vi "Init.vi"(8 "error in (no error)":errorcluster, 10 "Init Data":variant, 11 "Cryo Cooler in":refnum<class "Cryo Cooler.lvclass">) -> (0 "error out":errorcluster, 2 "Channel List":refnum<class "HK Item.lvclass">[](array[class]), 3 "Cryo Cooler out":refnum<class "Cryo Cooler.lvclass">)   [LabVIEW 2021, in "Cryo Cooler.lvclass"]
uses:
  Cryo Cooler.lvclass
  hk-channel-class/HK Item/HK Item.lvclass
  Cryo Cooler.lvclass/Cryo Cooler.ctl
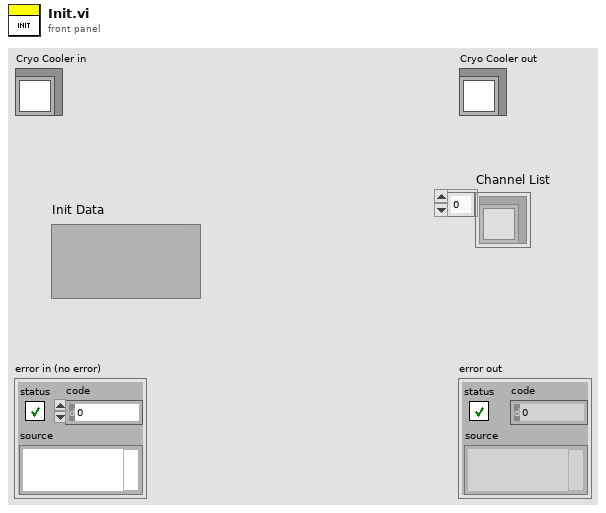
[diagram p1: front panel]
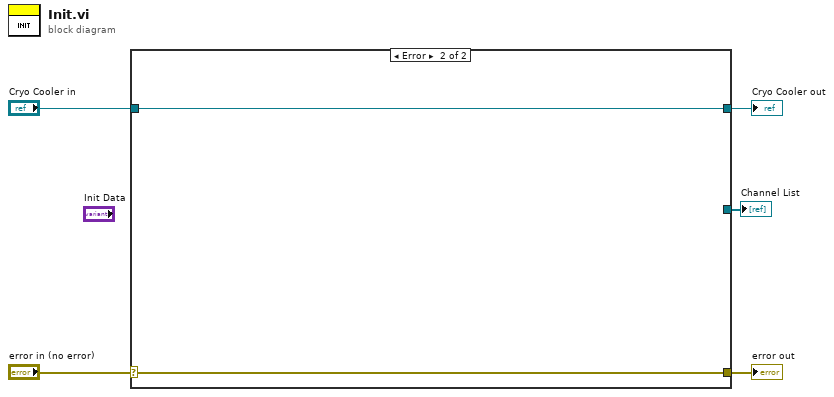
[diagram p0: block diagram]
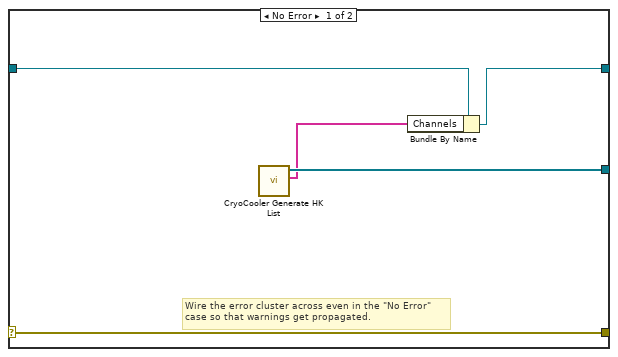
[diagram p2: hidden frame]
diagram:
  n1 = case shown="Error" "error in (no error)" {
    selector: "error in (no error)" -> [w10 w12]
    tunnel: [w10 w12] -> w4
    tunnel: [w7 w11] -> w2
    tunnel: "Cryo Cooler in" -> [w6 w11]
    tunnel: [w9 _] -> w1
    frame No Error {
      # "Wire the error cluster across even in the \"No Error\"\ncase so that warnings get propagated."
      n2 = call "CryoCooler Generate HK List.vi"() -> ("Channel Names"=w8:string[], "Channel List"=w9:refnum<class "HK Item.lvclass">[])  [unwired: 10 in]
      n3 = Bundle By Name(cluster=w6, "Channels"=w8) -> (w7:refnum<class "Cryo Cooler.lvclass">)
    }
    frame Error {
    }
  }
  "error out" <- w4
  "Cryo Cooler out" <- w2
  "Channel List" <- w1
